vi "Get-Set Histogram Fit Parameters.vi"(6 "Get(F)/Set":bool, 8 "Error In":errorcluster, 9 "Fixed Parameters":T4, 11 "Fit Settings":T1 {"Ramp Type" items=["Linear", "Logarithmic"]; "Fit Method" items=["Least Square", "Least Absolute Residual", "Bisquare"]}) -> (0 "Error Out":errorcluster, 1 "Fixed Parameters":T4, 3 "Fit Settings":T1 {"Ramp Type" items=["Linear", "Logarithmic"]; "Fit Method" items=["Least Square", "Least Absolute Residual", "Bisquare"]}, 4 "Initialized?":bool)   [LabVIEW 2019, in "Histogram Window.lvlib"]
uses:
  Histogram Window.lvlib
  D-Only Fixed Parameters.ctl
  Fit Settings.ctl
  <vilib>/Analysis/6fits.llb/Curve Fitting Criteria.ctl
  Ramp Type.ctl
  <vilib>/Analysis/NI_AALPro.lvlib
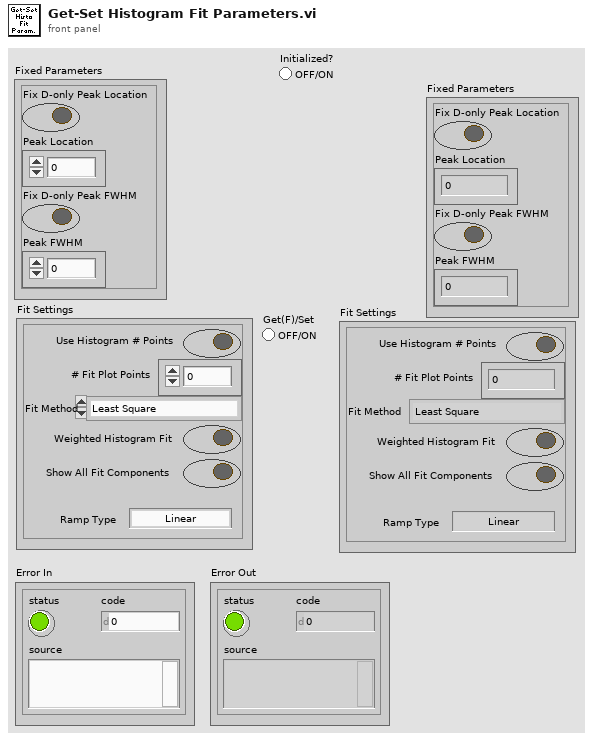
[diagram p1: front panel]
types:
  T1 = typedef "Fit Settings.ctl" = cluster{"Use Histogram # Points":bool, "# Fit Plot Points":u32, "Fit Method":T2, "Weighted Histogram Fit":bool, "Show All Fit Components":bool, "Ramp Type":T3}
  T2 = typedef "NI_AALPro.lvlib/Curve Fitting Criteria.ctl" = u16
  T3 = typedef "Ramp Type.ctl" = u16
  T4 = typedef "D-Only Fixed Parameters.ctl" = cluster{"Fix D-only Peak Location":bool, "Peak Location":dbl, "Fix D-only Peak FWHM":bool, "Peak FWHM":dbl}
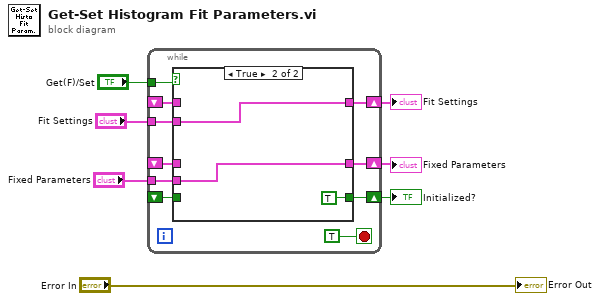
[diagram p0: block diagram]
diagram:
  n1 = while {
    tunnel: "Get(F)/Set" -> [w16]
    shift-right: [w14] -> w4
    shift-left: _ -> [w11]
    shift-right: [w13] -> w2
    shift-left: _ -> [w10]
    tunnel: "Fit Settings" -> [w15]
    tunnel: "Fixed Parameters" -> [w12]
    shift-right: [w9] -> w1
    shift-left: _ -> [w8]
    stop <- TRUE stop-if-true
    n2 = case shown="True" w16 {
      tunnel: w15 -> [_ w23]
      tunnel: [w20 w23] -> w14
      tunnel: [w19 w22] -> w13
      tunnel: w12 -> [_ w22]
      tunnel: w11 -> [w20 _]
      tunnel: w10 -> [w19 _]
      tunnel: [w18 TRUE] -> w9
      tunnel: w8 -> [w18 _]
      frame False {
      }
      frame True {
      }
    }
  }
  "Fixed Parameters" <- w2
  "Fit Settings" <- w4
  "Initialized?" <- w1
  "Error Out" <- "Error In"
